vi "Get Force Stand Status.vi"(8 "error in (no error)":errorcluster, 11 "ESM303 in":refnum<class "ESM303.lvclass">) -> (0 "error out":errorcluster, 2 "Status":variant, 3 "ESM303 out":refnum<class "ESM303.lvclass">)   [LabVIEW 2018, in "ESM303.lvlib" / "ESM303.lvclass"]
uses:
  ESM303.lvclass
  Custom Controls/Status.ctl
  builds/Force Test Stand/Force Test Stand/Force Test Stand.lvlibp/Force Test Stand.lvclass
  C:/Projects/LabVIEW/In-Progress/Jose Rivero-Diaz/builds/Force Test Stand/Force Test Stand/Force Test Stand.lvlibp/Force Test Stand.lvclass
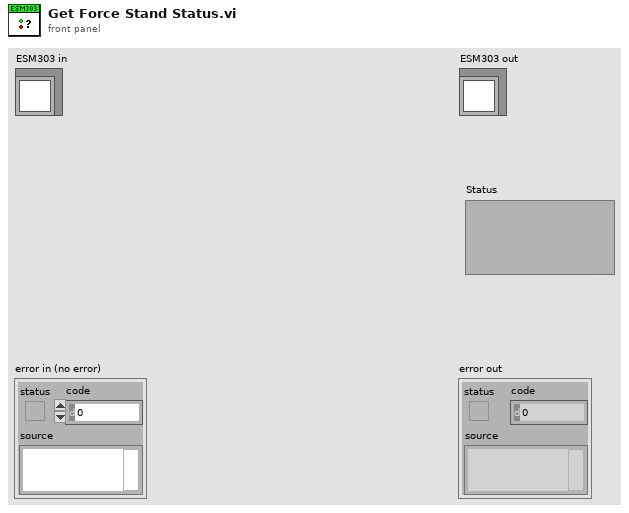
[diagram p1: front panel]
types:
  T1 = typedef "ESM303.lvlib/ESM303.lvclass/Status.ctl" = cluster{"Crosshead Status":string, "Operating Mode":string, "Limit Switch Status":string}
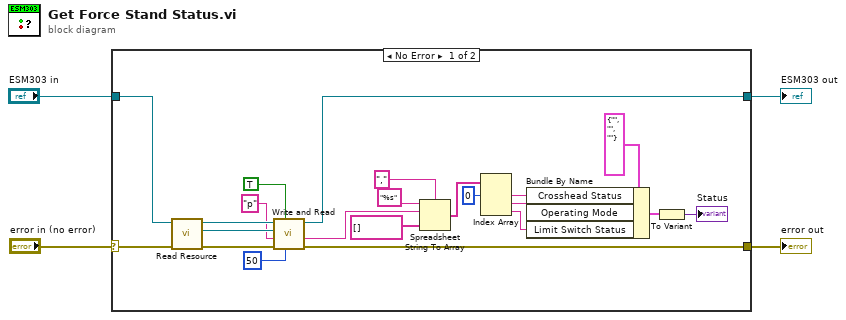
[diagram p0: block diagram]
diagram:
  n1 = case shown="No Error" "error in (no error)" {
    selector: "error in (no error)" -> [w26 w28]
    tunnel: [w18 w28] -> w3
    tunnel: [w17 w27] -> w2
    tunnel: "ESM303 in" -> [w25 w27]
    frame No Error {
      n2 = call "Read Resource.vi"("error in (no error)"=w26, "Force Test Stand in"=w25) -> ("error out"=w24:errorcluster, "Resource"=w21:refnum<visa-resource-name>, "Force Test Stand out"=w23:refnum<class "ESM303.lvclass">)  [unwired: 7 in]
      n3 = call "Write and Read.vi"("Delay Before Read (ms)"=50, "Write & Read"=TRUE, "error in (no error)"=w24, "Command"="p", "VISA Refnum in"=w21, "ESM303 in"=w23) -> ("error out"=w18:errorcluster, "Response"=w14:string, "ESM303 out"=w17:refnum<class "ESM303.lvclass">)  [unwired: 3 in]
      n4 = Spreadsheet String To Array(delimiter (Tab)=",", format string="%s", spreadsheet string=w14, array type (2D Dbl)=string[] []) -> (array=w12:string[])
      n5 = Index Array(array=w12, index #1=0 ("index")) -> (element #1=w9:string, element #2=w8:string, element #3=w7:string)  [unwired: 2 in]
      n6 = Bundle By Name(cluster=T1 {"Crosshead Status"="", "Operating Mode"="", "Limit Switch Status"=""} ("Status"), "Crosshead Status"=w9, "Operating Mode"=w8, "Limit Switch Status"=w7) -> (w6:T1)
      n7 = To Variant(anything=w6) -> (Variant=→"Status":variant)
    }
    frame Error {
    }
  }
  "error out" <- w3
  "ESM303 out" <- w2
